vi "Read Limit(String).vi"(8 "error in (no error)":errorcluster, 11 "Test":string) -> (0 "error out":errorcluster, 2 "a":string, 3 "b":string)   [LabVIEW 2019, in "Unit Test Engine Tools.lvlib"]
uses:
  Unit Test Engine Tools.lvlib
  LVUT Global 1.vi
  <vilib>/Utility/file.llb/Read Delimited Spreadsheet (string).vi
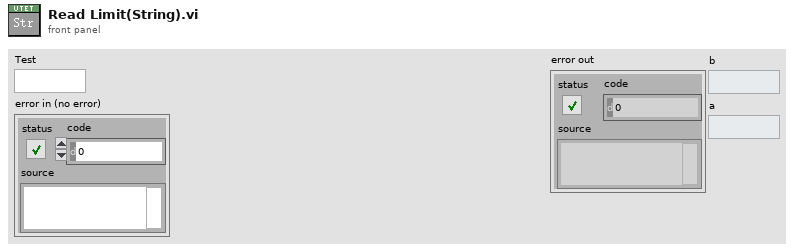
[diagram p1: front panel]
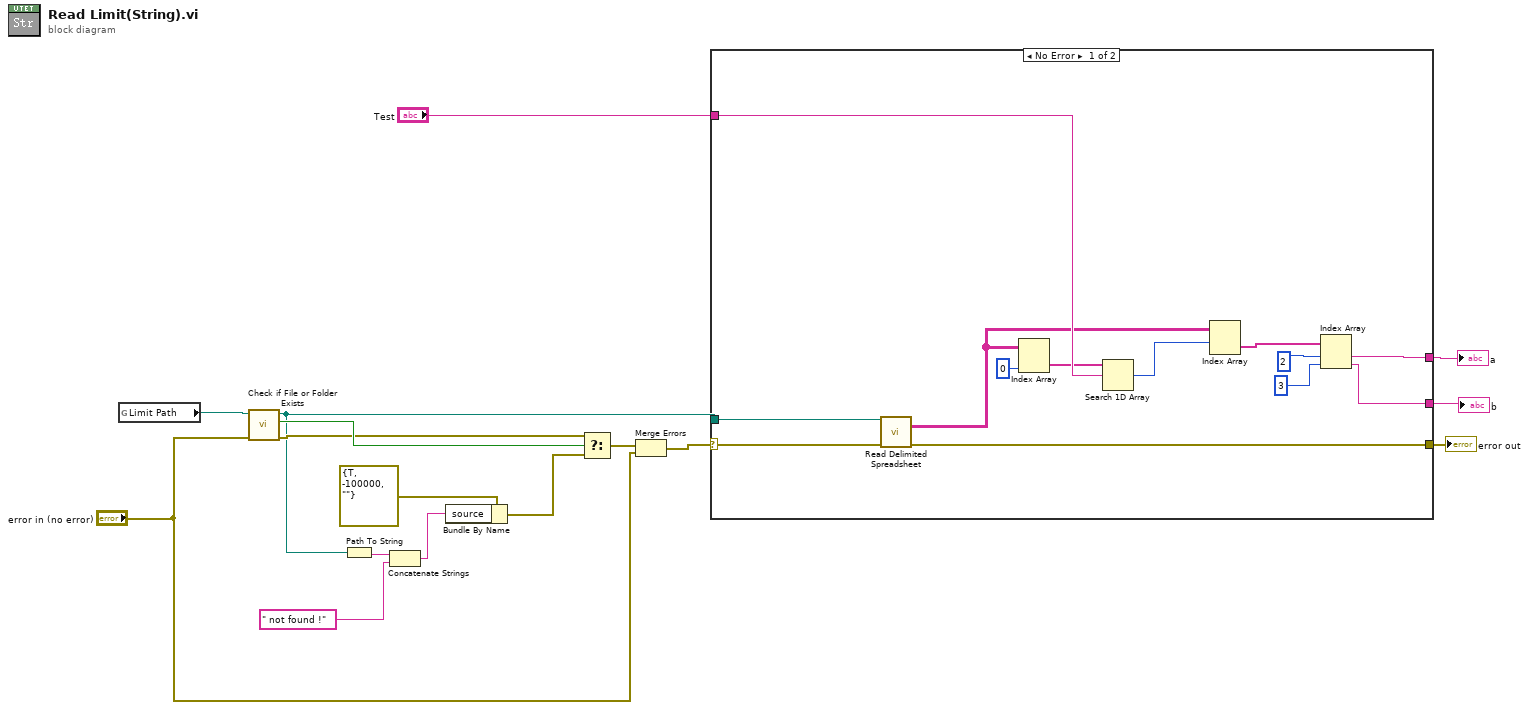
[diagram p0: block diagram]
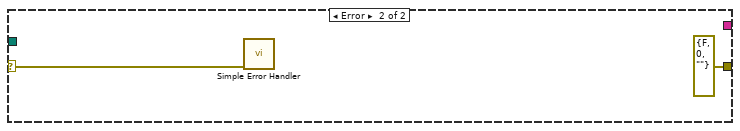
[diagram p2: hidden frame]
diagram:
  n1 = global read "LVUT Global 1.vi" "Limit Path"() -> (w12:path)
  n2 = call <vilib>:"Check if File or Folder Exists.vi"("error in (no error)"="error in (no error)", "path"=w12) -> ("error out"=w10:errorcluster, "file or folder exists?"=w11:bool, "dup path"=w5:path)  [unwired: 7 in]
  n3 = Path To String(path=w5) -> (string=w14:string)
  n4 = Concatenate Strings(w14, " not found !" ("string")) -> (w7:string)
  n5 = Bundle By Name(cluster=errorcluster {"status"=TRUE, "code"=-100000, "source"=""} ("f"), "source"=w7) -> (w8:errorcluster)
  n6 = Select(t=w10, s=w11, f=w8) -> (s? t:f=w6:errorcluster)
  n7 = Merge Errors(w6, "error in (no error)") -> (w4:errorcluster)
  n8 = case shown="No Error" w4 {
    selector: w4 -> [w18 w31]
    tunnel: "Test" -> [w29 _]
    tunnel: [w28 _] -> w2
    tunnel: [w27 _] -> w1
    tunnel: [w26 errorcluster {"status"=FALSE, "code"=0, "source"=""} ("error out")] -> w15
    tunnel: w5 -> [w17 _]
    frame No Error {
      n9 = call-poly <vilib>:"Read Delimited Spreadsheet.vi"("file path (dialog if empty)"=w17, "error in (no error)"=w18) -> ("all rows"=w23:string[][], "error out"=w26:errorcluster)  [unwired: 8 in, 4 out]
      n10 = Index Array(array=w23, index (col)=0 ("disabled index (col)")) -> (element=w24:string[])  [unwired: 1 in]
      n11 = Search 1D Array(1D array=w24, element=w29) -> (index of element=w22:i32)  [unwired: 1 in]
      n12 = Index Array(array=w23, index (row)=w22) -> (element=w21:string[])  [unwired: 1 in]
      n13 = Index Array(array=w21, index #1=2 ("index"), index #2=3 ("index")) -> (element #1=w28:string, element #2=w27:string)
    }
    frame Error {
      n14 = call <vilib>:"Simple Error Handler.vi"("error in (no error)"=w31) -> ()  [unwired: 4 in, 5 out]
    }
  }
  "error out" <- w15
  "b" <- w1
  "a" <- w2
